vi "To Pretty String (Boolean).vi"(7 "enable LabVIEW extensions? (T)":bool=TRUE, 8 "error in (no error)":errorcluster, 10 "indent":i32, 11 "JSON Value in":refnum<class "JSON Value.lvclass">) -> (0 "error out":errorcluster, 3 "String":string)   [LabVIEW 2016, in "JSON Value.lvclass"]
uses:
  JSON Value.lvclass
  JSON Value.lvclass/JSON Value.ctl
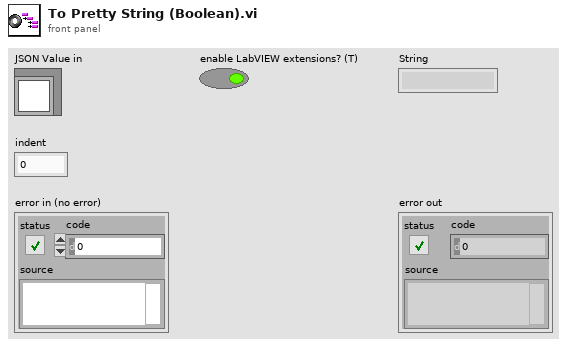
[diagram p1: front panel]
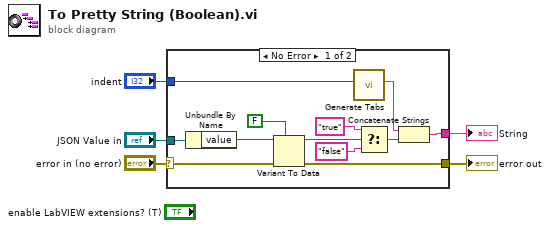
[diagram p0: block diagram]
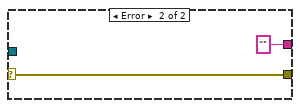
[diagram p2: hidden frame]
diagram:
  n1 = case shown="No Error" "error in (no error)" {
    selector: "error in (no error)" -> [w12 w18]
    tunnel: "JSON Value in" -> [w17 _]
    tunnel: [w6 "" ("f")] -> w4
    tunnel: [w11 w18] -> w2
    tunnel: "indent" -> [w9 _]
    frame No Error {
      n2 = Unbundle By Name(w17) -> ("value"=w16:variant)
      n3 = Variant To Data(error in=w12, type=FALSE, Variant=w16) -> (data=w10:bool, error out=w11:errorcluster)
      n4 = call "Generate Tabs.vi"("indent"=w9) -> ("Tabs"=w8:string)  [unwired: 9 in, 1 out]
      n5 = Select(t="true" ("String"), s=w10, f="false") -> (s? t:f=w7:string)
      n6 = Concatenate Strings(w8, w7) -> (w6:string)
    }
    frame Error {
    }
  }
  "String" <- w4
  "error out" <- w2
